vi "ChangeConfigGUI.vi"(4 "error in (no error)":errorcluster, 5 "Configuration Flags":T3, 6 "Configuration Read":T4 {"Select Mode:" items=["Custom", "Imaging", "300 All", "600 UV", "600 Blue", "600 Mid", "600 Red", "1200 m0", "1200 m1", "1200 m2", "1200 m3", "1200 m4", "1200 m5", "1200 m6", "1200 m7", "1200 RESOLVE", "400 m1", "400 m2", "930 m1", "930 m2", "930 m3", "930 m4", "930 m5", "930 m6", "400KL"]}, 7 "Alt Cam Focus":i32) -> (0 "error out":errorcluster, 1 "Script":T1[](array[typedef]), 2 "Targets":T2 {"Select Mode:" items=["Custom", "Imaging", "300 All", "600 UV", "600 Blue", "600 Mid", "600 Red", "1200 m0", "1200 m1", "1200 m2", "1200 m3", "1200 m4", "1200 m5", "1200 m6", "1200 m7", "1200 RESOLVE", "400 m1", "400 m2", "930 m1", "930 m2", "930 m3", "930 m4", "930 m5", "930 m6", "400KL"]})   [LabVIEW 2015]
doc: "This GUI interprets supplied configuration information and displays it to the user. It compares the target configuration to the machine state (what components are loaded) and checks for compatibility. If the user choses to start a move, an enumerated script is output that can be used to start a sequence of moves."
uses:
  GSP_ObsConfig.llb/configuration.ctl
  Script_actions.ctl
  Users/Stephen/Desktop/BETA_GSCS - Copy/Dialog/dialog_messages.ctl
  Users/Stephen/Desktop/BETA_GSCS - Copy/GUI/GSP_GUI_global.vi
panel:
  in  "Something not loaded?":bool
  out "Date":string
  out "User":string
  out "Name":string
  in  "Start Move":bool
  in  "Configuration":i32(listbox)
  # "Systems will finish any current scripts \nbefore beginning the configuration\nchange."
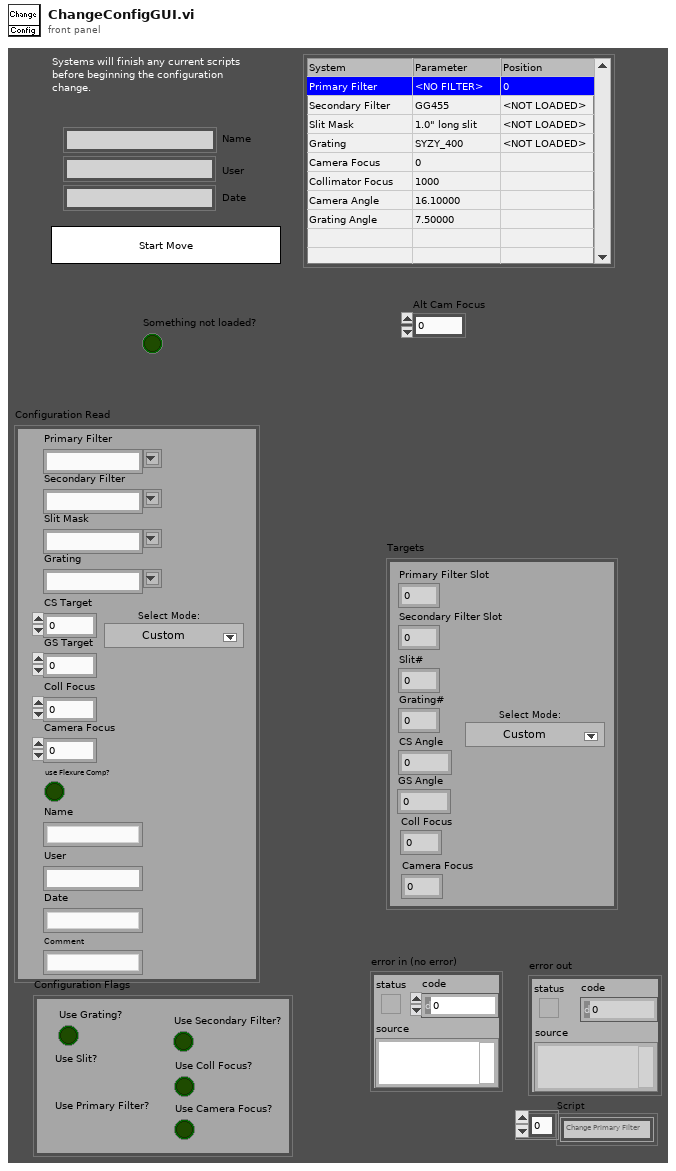
[diagram p1: front panel]
types:
  T1 = typedef "Script_actions.ctl" = enum16{"Change Primary Filter", "Change Secondary Filter", "Change Collimator Focus", "Change Camera Focus", "Change Grating", "Change Angles", "Change Slit Mask", "Toggle Slit", "Change WAVMODE", "Check All Systems", "Change Flexure"}
  T2 = cluster{"Primary Filter Slot":i32, "Secondary Filter Slot":i32, "Slit#":i32, "Grating#":i32, "CS Angle":dbl, "GS Angle":dbl, "Coll Focus":i32, "Camera Focus":i32, "Select Mode:":u16}
  T3 = cluster{"Use Grating?":bool, "Use Slit?":bool, "Use Primary Filter?":bool, "Use Secondary Filter?":bool, "Use Coll Focus?":bool, "Use Camera Focus?":bool}
  T4 = typedef "configuration.ctl" = cluster{"Primary Filter":string, "Secondary Filter":string, "Slit Mask":string, "Grating":string, "CS Target":dbl, "GS Target":dbl, "Coll Focus":i32, "Camera Focus":i32, "Name":string, "User":string, "Date":string, "Comment":string, "use Flexure Comp?":bool, "Select Mode:":u16}
  T5 = cluster{"Primary Filter Slot":i32, "Secondary Filter Slot":i32, "Slit#":i32, "Grating#":i32, "CS Angle":dbl, "GS Angle":dbl, "Coll Focus":i32, "Camera Focus":i32, "Select Mode":i32}
  T6 = typedef "dialog_messages.ctl" = enum16{"Custom", "Incompatible Config"}
  T7 = cluster{"Grating#":i32, "Slit#":i32, "Primary Filter#":i32, "Secondary Filter#":i32, "Coll Position":i32, "Camera Focus":i32, "Camera Angle":dbl, "Grating Angle":dbl, "Coll Temp":dbl, "CF Temp\n":dbl, "Camera Target":dbl, "Grating Target":dbl, "WAVMODE":string, "Slit Hidden??":bool}
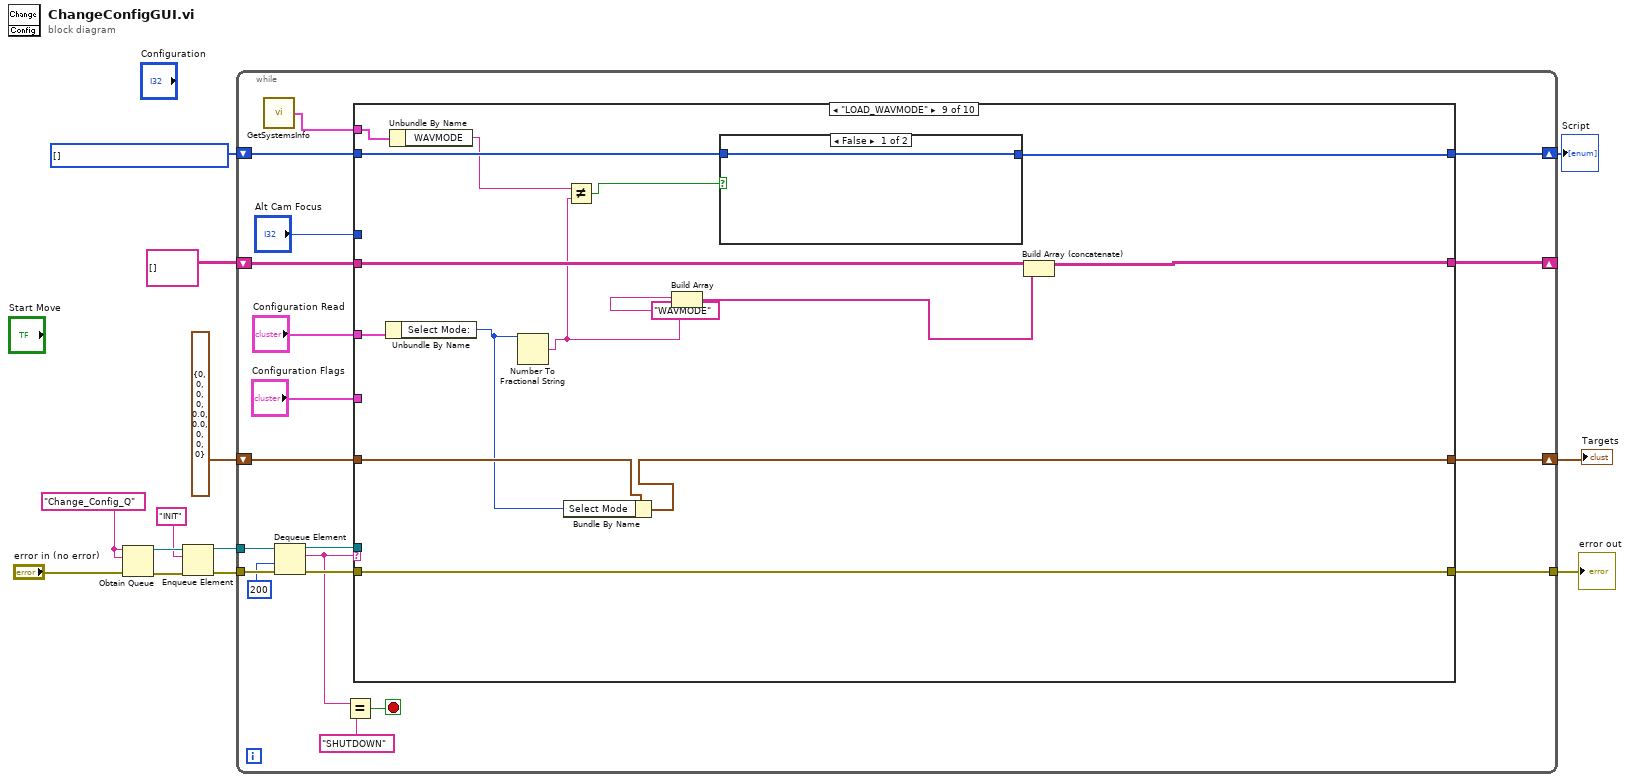
[diagram p0: block diagram]
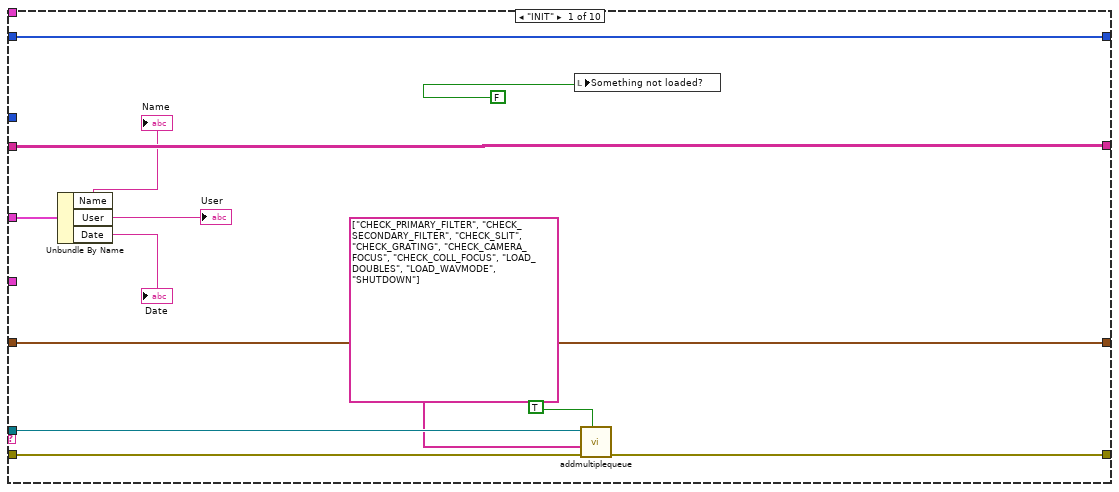
[diagram p2: hidden frame]
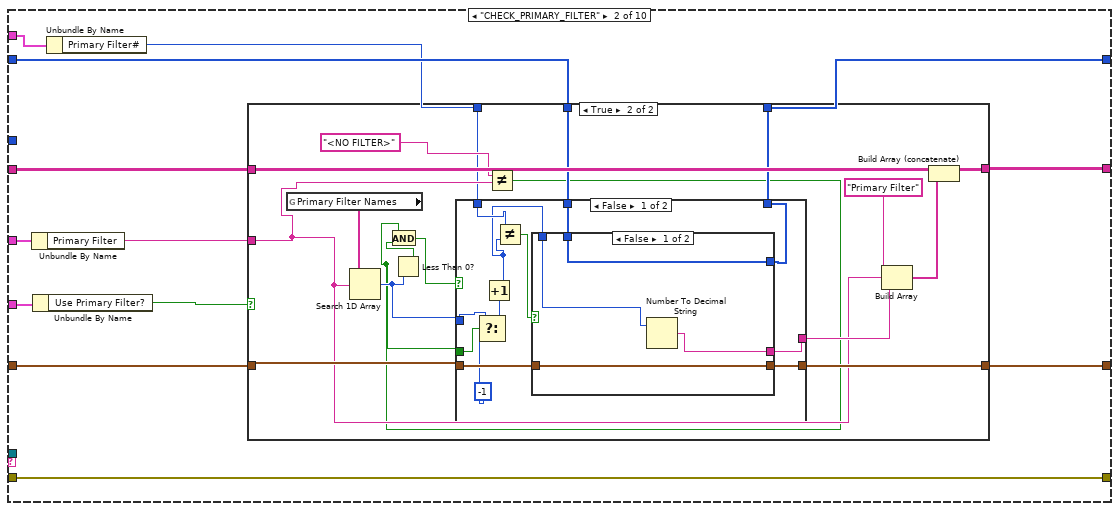
[diagram p3: hidden frame]
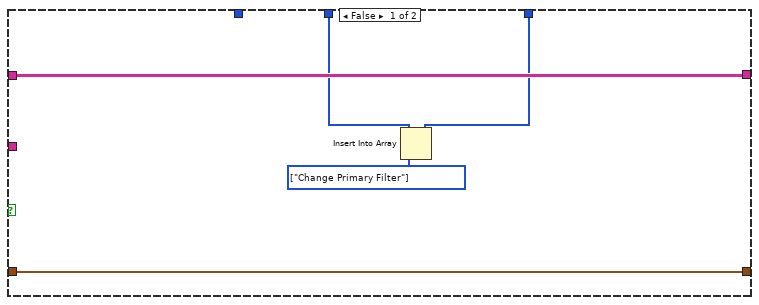
[diagram p4: hidden frame]
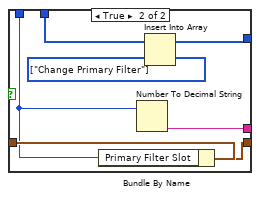
[diagram p5: hidden frame]
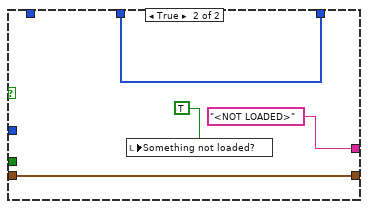
[diagram p6: hidden frame]
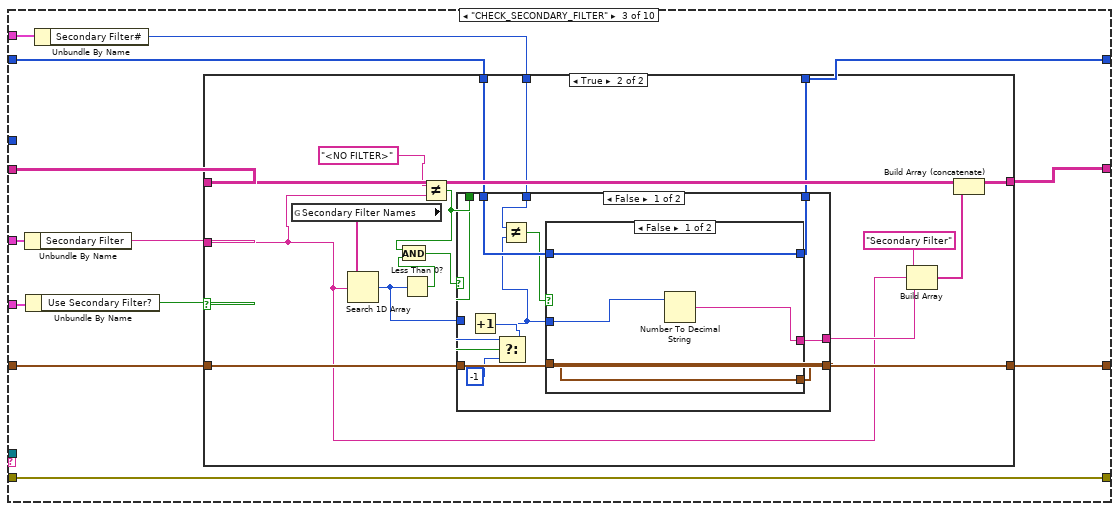
[diagram p7: hidden frame]
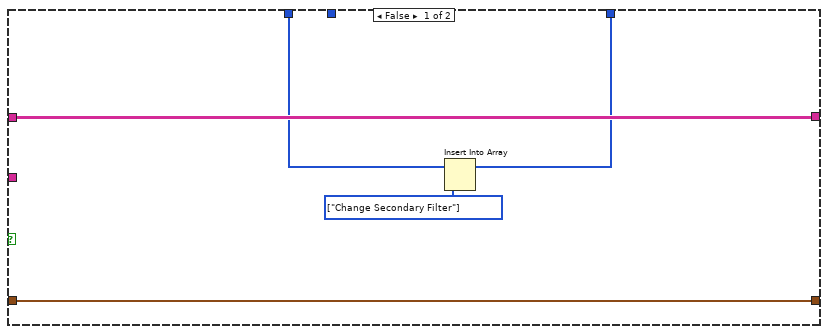
[diagram p8: hidden frame]
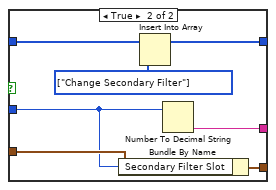
[diagram p9: hidden frame]
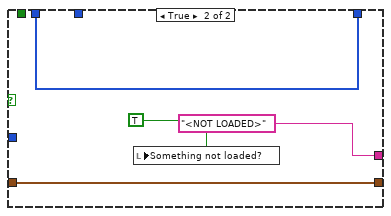
[diagram p10: hidden frame]
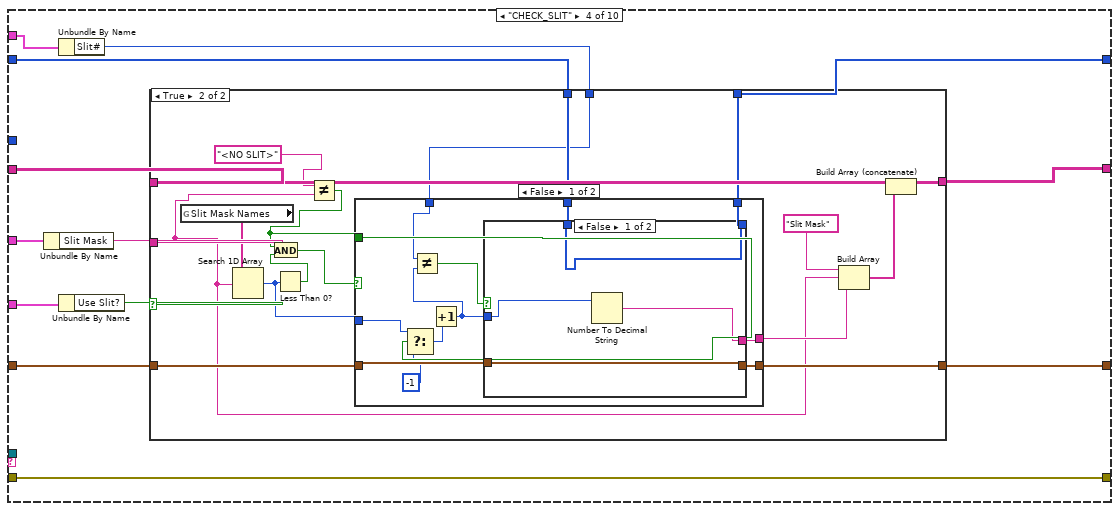
[diagram p11: hidden frame]
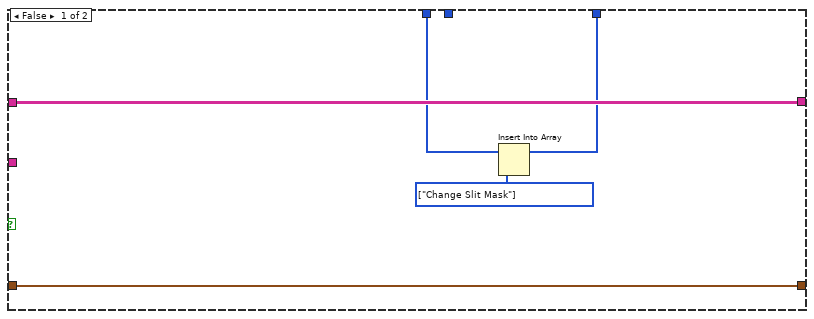
[diagram p12: hidden frame]
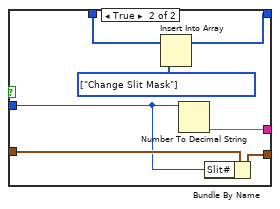
[diagram p13: hidden frame]
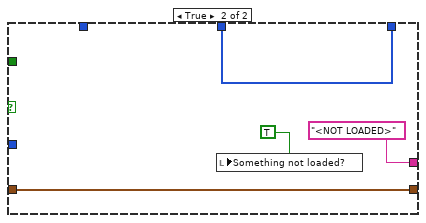
[diagram p14: hidden frame]
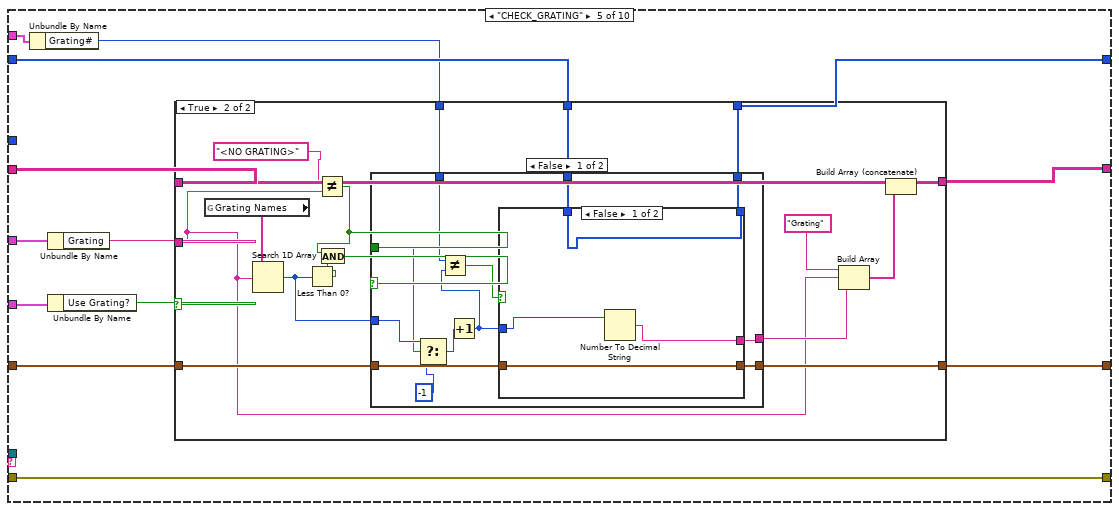
[diagram p15: hidden frame]
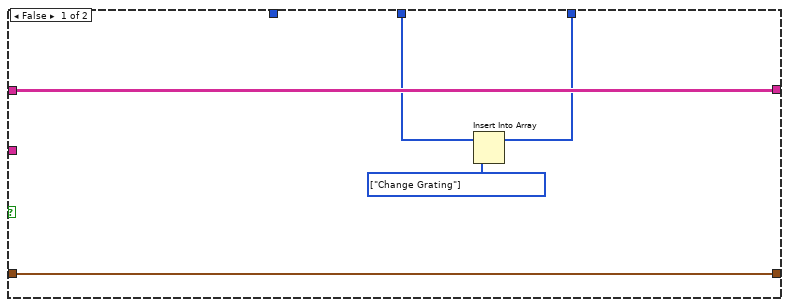
[diagram p16: hidden frame]
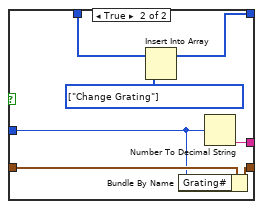
[diagram p17: hidden frame]
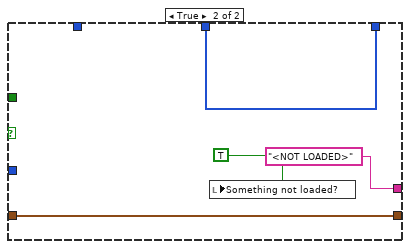
[diagram p18: hidden frame]
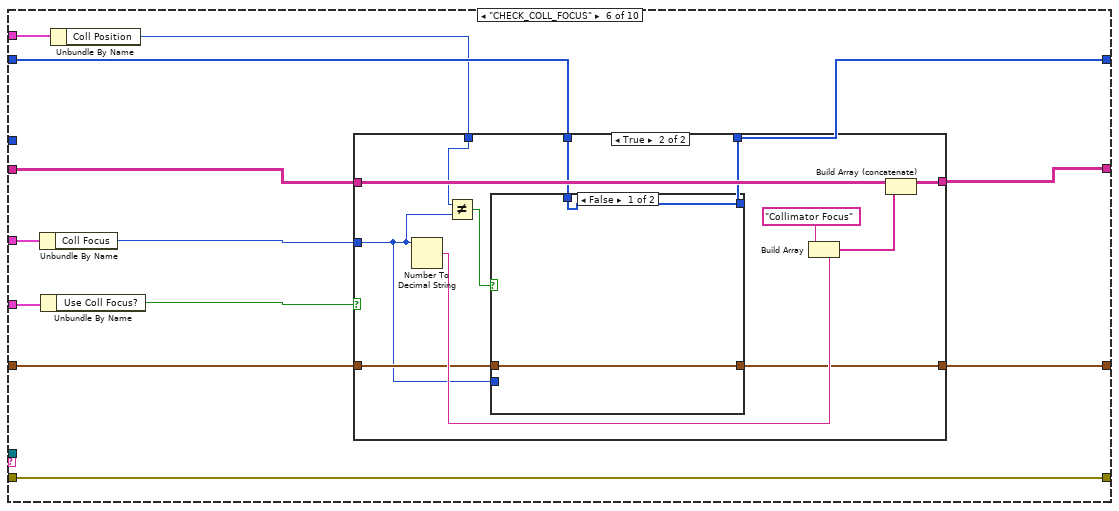
[diagram p19: hidden frame]
diagram:
  w4 = T1[] [] items=["Change Primary Filter", "Change Secondary Filter", "Change Collimator Focus", "Change Camera Focus", "Change Grating", "Change Angles", "Change Slit Mask", "Toggle Slit", "Change WAVMODE", "Check All Systems", "Change Flexure"]
  w11 = "Change_Config_Q" ("name (unnamed)")
  n1 = Obtain Queue(name (unnamed)=w11, element data type=w11, error in (no error)="error in (no error)") -> (queue out=w8:refnum<queue>, error out=w9:errorcluster)  [unwired: 2 in, 1 out]
  n2 = Enqueue Element(queue=w8, element="INIT", error in (no error)=w9) -> (queue out=w7:refnum<queue>, error out=w10:errorcluster)  [unwired: 1 in, 1 out]
  n3 = while {
    tunnel: w10 -> [w31]
    tunnel: [w32] -> w13
    tunnel: w7 -> [w29]
    shift-right: [w22] -> _
    shift-left: string[][] [] -> [w23]
    shift-right: [w18] -> w1
    shift-left: w4 -> [w19]
    shift-right: [w16] -> w2
    shift-left: T5 {"Primary Filter Slot"=0, "Secondary Filter Slot"=0, "Slit#"=0, "Grating#"=0, "CS Angle"=0.0, "GS Angle"=0.0, "Coll Focus"=0, "Camera Focus"=0, "Select Mode"=0} ("Targets") -> [w17]
    stop <- w25 stop-if-true
    n4 = call "GetSystemsInfo.vi"() -> ("Pos Info"=w14:T7)
    n5 = Dequeue Element(queue=w29, timeout in ms (-1)=200, error in (no error)=w31) -> (queue out=w28:refnum<queue>, element=w27:string, error out=w30:errorcluster)  [unwired: 1 out]
    n6 = Equal?(x=w27, y="SHUTDOWN") -> (x = y?=w25:bool)
    n7 = case shown="\"LOAD_WAVMODE\"" w27 {
      tunnel: w30 -> [w40 w52 w114 w176 w238 w300 w340 w383 w427 w440]
      tunnel: [w38 w52 w114 w176 w238 w300 w340 w377 w427 w440] -> w32
      tunnel: w28 -> [w39 _ _ _ _ _ _ _ _ _]
      tunnel: w23 -> [w45 w56 w118 w180 w242 w304 w343 w391 w432 w439]
      tunnel: [w45 w53 w115 w177 w239 w301 w341 w382 w430 w439] -> w22
      tunnel: "Configuration Read" -> [w44 w58 w120 w182 w244 w306 w345 w386 w425 _]
      tunnel: "Configuration Flags" -> [_ w57 w119 w181 w243 w305 w344 _ _ _]
      tunnel: w19 -> [w36 w51 w113 w175 w237 w299 w339 w381 w429 w437]
      tunnel: [w36 w50 w112 w174 w236 w298 w338 w380 w428 w437] -> w18
      tunnel: w17 -> [w35 w49 w111 w173 w235 w297 w337 w385 w424 w438]
      tunnel: [w35 w48 w110 w172 w234 w296 w336 w384 w423 w438] -> w16
      tunnel: "Alt Cam Focus" -> [_ _ _ _ _ _ w333 _ _ _]
      tunnel: w14 -> [_ w47 w109 w171 w233 w295 w331 w376 w421 _]
      frame "INIT" {
        n8 = Unbundle By Name(w44) -> ("Name"=→"Name":string, "User"=→"User":string, "Date"=→"Date":string)
        n9 = local write "Something not loaded?"(FALSE) -> ()
        n10 = call "addmultiplequeue.vi"("Add All (false)"=TRUE, "error in (no error)"=w40, "Strings to Add"=string[] ["CHECK_PRIMARY_FILTER", "CHECK_SECONDARY_FILTER", "CHECK_SLIT", "CHECK_GRATING", "CHECK_CAMERA_FOCUS", "CHECK_COLL_FOCUS", "LOAD_DOUBLES", "LOAD_WAVMODE", "SHUTDOWN"], "queue"=w39) -> ("error out"=w38:errorcluster)  [unwired: 3 in, 1 out]
      }
      frame "CHECK_PRIMARY_FILTER" {
        n11 = Unbundle By Name(w58) -> ("Primary Filter"=w54:string)
        n12 = Unbundle By Name(w57) -> ("Use Primary Filter?"=w55:bool)
        n13 = Unbundle By Name(w47) -> ("Primary Filter#"=w46:i32)
        n14 = case shown="True" w55 {
          tunnel: w56 -> [w63 w77]
          tunnel: w54 -> [_ w68]
          tunnel: [w63 w78] -> w53
          tunnel: w51 -> [w62 w73]
          tunnel: [w61 w72] -> w50
          tunnel: w49 -> [w60 w71]
          tunnel: [w60 w70] -> w48
          tunnel: w46 -> [_ w64]
          frame False {
            w59 = T1[] [enum."Change Primary Filter"] items=["Change Primary Filter", "Change Secondary Filter", "Change Collimator Focus", "Change Camera Focus", "Change Grating", "Change Angles", "Change Slit Mask", "Toggle Slit", "Change WAVMODE", "Check All Systems", "Change Flexure"]
            n15 = Insert Into Array(array=w62, new element=w59) -> (w61:T1[])  [unwired: 1 in]
          }
          frame True {
            n16 = global read "GSP_GUI_global.vi" "Primary Filter Names"() -> (w80:string[])
            n17 = Search 1D Array(1D array=w80, element=w68) -> (index of element=w79:i32)  [unwired: 1 in]
            n18 = Less Than 0?(x=w79) -> (x < 0?=w67:bool)
            n19 = Not Equal?(x="<NO FILTER>", y=w68) -> (x != y?=w65:bool)
            n20 = And(x=w65, y=w67) -> (x .and. y?=w66:bool)
            n21 = case shown="False" w66 {
              tunnel: w79 -> [w86 _]
              tunnel: [w92 "<NOT LOADED>"] -> w75
              tunnel: w73 -> [w91 w106]
              tunnel: [w90 w106] -> w72
              tunnel: w71 -> [w89 w105]
              tunnel: [w88 w105] -> w70
              tunnel: w65 -> [w84 _]
              tunnel: w64 -> [w83 _]
              frame False {
                n22 = Select(t=w86, s=w84, f=-1) -> (s? t:f=w85:i32)
                n23 = Increment(x=w85) -> (x+1=w81:i32)
                n24 = Not Equal?(x=w83, y=w81) -> (x != y?=w82:bool)
                n25 = case shown="False" w82 {
                  tunnel: [w93 w103] -> w92
                  tunnel: w91 -> [w96 w102]
                  tunnel: [w96 w101] -> w90
                  tunnel: w89 -> [w95 w100]
                  tunnel: [w95 w99] -> w88
                  tunnel: w81 -> [w94 w98]
                  frame False {
                    n26 = Number To Decimal String(number=w94) -> (decimal integer string=w93:string)  [unwired: 1 in]
                  }
                  frame True {
                    w97 = T1[] [enum."Change Primary Filter"] items=["Change Primary Filter", "Change Secondary Filter", "Change Collimator Focus", "Change Camera Focus", "Change Grating", "Change Angles", "Change Slit Mask", "Toggle Slit", "Change WAVMODE", "Check All Systems", "Change Flexure"]
                    n27 = Bundle By Name(cluster=w100, "Primary Filter Slot"=w98) -> (w99:T5)
                    n28 = Number To Decimal String(number=w98) -> (decimal integer string=w103:string)  [unwired: 1 in]
                    n29 = Insert Into Array(array=w102, new element=w97) -> (w101:T1[])  [unwired: 1 in]
                  }
                }
              }
              frame True {
                n30 = local write "Something not loaded?"(TRUE) -> ()
              }
            }
            n31 = Build Array("Primary Filter", w68, w75) -> (w74:string[])
            n32 = Build Array (concatenate)(w77, w74) -> (w78:string[][])
          }
        }
      }
      frame "CHECK_SECONDARY_FILTER" {
        n33 = Unbundle By Name(w120) -> ("Secondary Filter"=w116:string)
        n34 = Unbundle By Name(w119) -> ("Use Secondary Filter?"=w117:bool)
        n35 = Unbundle By Name(w109) -> ("Secondary Filter#"=w108:i32)
        n36 = case shown="True" w117 {
          tunnel: w118 -> [w125 w139]
          tunnel: w116 -> [_ w130]
          tunnel: [w125 w140] -> w115
          tunnel: w113 -> [w124 w135]
          tunnel: [w123 w134] -> w112
          tunnel: w111 -> [w122 w133]
          tunnel: [w122 w132] -> w110
          tunnel: w108 -> [_ w126]
          frame False {
            w121 = T1[] [enum."Change Secondary Filter"] items=["Change Primary Filter", "Change Secondary Filter", "Change Collimator Focus", "Change Camera Focus", "Change Grating", "Change Angles", "Change Slit Mask", "Toggle Slit", "Change WAVMODE", "Check All Systems", "Change Flexure"]
            n37 = Insert Into Array(array=w124, new element=w121) -> (w123:T1[])  [unwired: 1 in]
          }
          frame True {
            n38 = global read "GSP_GUI_global.vi" "Secondary Filter Names"() -> (w142:string[])
            n39 = Search 1D Array(1D array=w142, element=w130) -> (index of element=w141:i32)  [unwired: 1 in]
            n40 = Less Than 0?(x=w141) -> (x < 0?=w129:bool)
            n41 = Not Equal?(x="<NO FILTER>", y=w130) -> (x != y?=w127:bool)
            n42 = And(x=w127, y=w129) -> (x .and. y?=w128:bool)
            n43 = case shown="False" w128 {
              tunnel: w141 -> [w148 _]
              tunnel: [w154 "<NOT LOADED>"] -> w137
              tunnel: w135 -> [w153 w168]
              tunnel: [w152 w168] -> w134
              tunnel: w133 -> [w151 w167]
              tunnel: [w150 w167] -> w132
              tunnel: w127 -> [w146 _]
              tunnel: w126 -> [w145 _]
              frame False {
                n44 = Select(t=w148, s=w146, f=-1) -> (s? t:f=w147:i32)
                n45 = Increment(x=w147) -> (x+1=w144:i32)
                n46 = Not Equal?(x=w145, y=w144) -> (x != y?=w143:bool)
                n47 = case shown="False" w143 {
                  tunnel: [w157 w165] -> w154
                  tunnel: w153 -> [w155 w164]
                  tunnel: [w155 w163] -> w152
                  tunnel: w151 -> [w156 w162]
                  tunnel: [w156 w161] -> w150
                  tunnel: w144 -> [w158 w160]
                  frame False {
                    n48 = Number To Decimal String(number=w158) -> (decimal integer string=w157:string)  [unwired: 1 in]
                  }
                  frame True {
                    w159 = T1[] [enum."Change Secondary Filter"] items=["Change Primary Filter", "Change Secondary Filter", "Change Collimator Focus", "Change Camera Focus", "Change Grating", "Change Angles", "Change Slit Mask", "Toggle Slit", "Change WAVMODE", "Check All Systems", "Change Flexure"]
                    n49 = Bundle By Name(cluster=w162, "Secondary Filter Slot"=w160) -> (w161:T5)
                    n50 = Insert Into Array(array=w164, new element=w159) -> (w163:T1[])  [unwired: 1 in]
                    n51 = Number To Decimal String(number=w160) -> (decimal integer string=w165:string)  [unwired: 1 in]
                  }
                }
              }
              frame True {
                n52 = local write "Something not loaded?"(TRUE) -> ()
              }
            }
            n53 = Build Array("Secondary Filter", w130, w137) -> (w136:string[])
            n54 = Build Array (concatenate)(w139, w136) -> (w140:string[][])
          }
        }
      }
      frame "CHECK_SLIT" {
        n55 = Unbundle By Name(w182) -> ("Slit Mask"=w178:string)
        n56 = Unbundle By Name(w171) -> ("Slit#"=w170:i32)
        n57 = Unbundle By Name(w181) -> ("Use Slit?"=w179:bool)
        n58 = case shown="True" w179 {
          tunnel: w180 -> [w187 w201]
          tunnel: w178 -> [_ w192]
          tunnel: [w187 w202] -> w177
          tunnel: w175 -> [w186 w197]
          tunnel: [w185 w196] -> w174
          tunnel: w173 -> [w184 w195]
          tunnel: [w184 w194] -> w172
          tunnel: w170 -> [_ w188]
          frame False {
            w183 = T1[] [enum."Change Slit Mask"] items=["Change Primary Filter", "Change Secondary Filter", "Change Collimator Focus", "Change Camera Focus", "Change Grating", "Change Angles", "Change Slit Mask", "Toggle Slit", "Change WAVMODE", "Check All Systems", "Change Flexure"]
            n59 = Insert Into Array(array=w186, new element=w183) -> (w185:T1[])  [unwired: 1 in]
          }
          frame True {
            n60 = global read "GSP_GUI_global.vi" "Slit Mask Names"() -> (w204:string[])
            n61 = Search 1D Array(1D array=w204, element=w192) -> (index of element=w203:i32)  [unwired: 1 in]
            n62 = Less Than 0?(x=w203) -> (x < 0?=w191:bool)
            n63 = Not Equal?(x="<NO SLIT>", y=w192) -> (x != y?=w189:bool)
            n64 = And(x=w189, y=w191) -> (x .and. y?=w190:bool)
            n65 = case shown="False" w190 {
              tunnel: w203 -> [w211 _]
              tunnel: [w216 "<NOT LOADED>"] -> w199
              tunnel: w197 -> [w215 w230]
              tunnel: [w214 w230] -> w196
              tunnel: w195 -> [w213 w229]
              tunnel: [w212 w229] -> w194
              tunnel: w189 -> [w210 _]
              tunnel: w188 -> [w206 _]
              frame False {
                n66 = Select(t=w211, s=w210, f=-1) -> (s? t:f=w208:i32)
                n67 = Increment(x=w208) -> (x+1=w207:i32)
                n68 = Not Equal?(x=w206, y=w207) -> (x != y?=w205:bool)
                n69 = case shown="False" w205 {
                  tunnel: [w219 w227] -> w216
                  tunnel: w215 -> [w217 w226]
                  tunnel: [w217 w225] -> w214
                  tunnel: w213 -> [w218 w224]
                  tunnel: [w218 w223] -> w212
                  tunnel: w207 -> [w220 w222]
                  frame False {
                    n70 = Number To Decimal String(number=w220) -> (decimal integer string=w219:string)  [unwired: 1 in]
                  }
                  frame True {
                    w221 = T1[] [enum."Change Slit Mask"] items=["Change Primary Filter", "Change Secondary Filter", "Change Collimator Focus", "Change Camera Focus", "Change Grating", "Change Angles", "Change Slit Mask", "Toggle Slit", "Change WAVMODE", "Check All Systems", "Change Flexure"]
                    n71 = Insert Into Array(array=w226, new element=w221) -> (w225:T1[])  [unwired: 1 in]
                    n72 = Number To Decimal String(number=w222) -> (decimal integer string=w227:string)  [unwired: 1 in]
                    n73 = Bundle By Name(cluster=w224, "Slit#"=w222) -> (w223:T5)
                  }
                }
              }
              frame True {
                n74 = local write "Something not loaded?"(TRUE) -> ()
              }
            }
            n75 = Build Array("Slit Mask", w192, w199) -> (w198:string[])
            n76 = Build Array (concatenate)(w201, w198) -> (w202:string[][])
          }
        }
      }
      frame "CHECK_GRATING" {
        n77 = Unbundle By Name(w233) -> ("Grating#"=w232:i32)
        n78 = Unbundle By Name(w244) -> ("Grating"=w240:string)
        n79 = Unbundle By Name(w243) -> ("Use Grating?"=w241:bool)
        n80 = case shown="True" w241 {
          tunnel: w242 -> [w249 w263]
          tunnel: w240 -> [_ w253]
          tunnel: [w249 w264] -> w239
          tunnel: w237 -> [w248 w259]
          tunnel: [w247 w258] -> w236
          tunnel: w235 -> [w246 w257]
          tunnel: [w246 w256] -> w234
          tunnel: w232 -> [_ w250]
          frame False {
            w245 = T1[] [enum."Change Grating"] items=["Change Primary Filter", "Change Secondary Filter", "Change Collimator Focus", "Change Camera Focus", "Change Grating", "Change Angles", "Change Slit Mask", "Toggle Slit", "Change WAVMODE", "Check All Systems", "Change Flexure"]
            n81 = Insert Into Array(array=w248, new element=w245) -> (w247:T1[])  [unwired: 1 in]
          }
          frame True {
            n82 = global read "GSP_GUI_global.vi" "Grating Names"() -> (w266:string[])
            n83 = Search 1D Array(1D array=w266, element=w253) -> (index of element=w265:i32)  [unwired: 1 in]
            n84 = Less Than 0?(x=w265) -> (x < 0?=w255:bool)
            n85 = Not Equal?(x="<NO GRATING>", y=w253) -> (x != y?=w251:bool)
            n86 = And(x=w251, y=w255) -> (x .and. y?=w254:bool)
            n87 = case shown="False" w254 {
              tunnel: w265 -> [w272 _]
              tunnel: [w278 "<NOT LOADED>"] -> w261
              tunnel: w259 -> [w277 w292]
              tunnel: [w276 w292] -> w258
              tunnel: w257 -> [w275 w291]
              tunnel: [w274 w291] -> w256
              tunnel: w251 -> [w270 _]
              tunnel: w250 -> [w267 _]
              frame False {
                n88 = Select(t=w272, s=w270, f=-1) -> (s? t:f=w271:i32)
                n89 = Increment(x=w271) -> (x+1=w268:i32)
                n90 = Not Equal?(x=w267, y=w268) -> (x != y?=w269:bool)
                n91 = case shown="False" w269 {
                  tunnel: [w279 w289] -> w278
                  tunnel: w277 -> [w282 w288]
                  tunnel: [w282 w287] -> w276
                  tunnel: w275 -> [w281 w286]
                  tunnel: [w281 w285] -> w274
                  tunnel: w268 -> [w280 w284]
                  frame False {
                    n92 = Number To Decimal String(number=w280) -> (decimal integer string=w279:string)  [unwired: 1 in]
                  }
                  frame True {
                    w283 = T1[] [enum."Change Grating"] items=["Change Primary Filter", "Change Secondary Filter", "Change Collimator Focus", "Change Camera Focus", "Change Grating", "Change Angles", "Change Slit Mask", "Toggle Slit", "Change WAVMODE", "Check All Systems", "Change Flexure"]
                    n93 = Insert Into Array(array=w288, new element=w283) -> (w287:T1[])  [unwired: 1 in]
                    n94 = Bundle By Name(cluster=w286, "Grating#"=w284) -> (w285:T5)
                    n95 = Number To Decimal String(number=w284) -> (decimal integer string=w289:string)  [unwired: 1 in]
                  }
                }
              }
              frame True {
                n96 = local write "Something not loaded?"(TRUE) -> ()
              }
            }
            n97 = Build Array("Grating", w253, w261) -> (w260:string[])
            n98 = Build Array (concatenate)(w263, w260) -> (w264:string[][])
          }
        }
      }
      frame "CHECK_COLL_FOCUS" {
        n99 = Unbundle By Name(w306) -> ("Coll Focus"=w302:i32)
        n100 = Unbundle By Name(w305) -> ("Use Coll Focus?"=w303:bool)
        n101 = Unbundle By Name(w295) -> ("Coll Position"=w294:i32)
        n102 = case shown="True" w303 {
          tunnel: w304 -> [w309 w320]
          tunnel: w302 -> [_ w311]
          tunnel: [w309 w321] -> w301
          tunnel: w299 -> [w307 w317]
          tunnel: [w307 w316] -> w298
          tunnel: w297 -> [w308 w314]
          tunnel: [w308 w313] -> w296
          tunnel: w294 -> [_ w312]
          frame False {
          }
          frame True {
            n103 = Number To Decimal String(number=w311) -> (decimal integer string=w315:string)  [unwired: 1 in]
            n104 = Not Equal?(x=w312, y=w311) -> (x != y?=w310:bool)
            n105 = case shown="False" w310 {
              tunnel: w317 -> [w323 w329]
              tunnel: [w323 w328] -> w316
              tunnel: w314 -> [w322 w327]
              tunnel: w311 -> [_ w326]
              tunnel: [w322 w325] -> w313
              frame False {
              }
              frame True {
                w324 = T1[] [enum."Change Collimator Focus"] items=["Change Primary Filter", "Change Secondary Filter", "Change Collimator Focus", "Change Camera Focus", "Change Grating", "Change Angles", "Change Slit Mask", "Toggle Slit", "Change WAVMODE", "Check All Systems", "Change Flexure"]
                n106 = Bundle By Name(cluster=w327, "Coll Focus"=w326) -> (w325:T5)
                n107 = Insert Into Array(array=w329, new element=w324) -> (w328:T1[])  [unwired: 1 in]
              }
            }
            n108 = Build Array("Collimator Focus", w315) -> (w318:string[])
            n109 = Build Array (concatenate)(w320, w318) -> (w321:string[][])
          }
        }
      }
      frame "CHECK_CAMERA_FOCUS" {
        n110 = Not Equal To 0?(x=w333) -> (x != 0?=w334:bool)
        n111 = Unbundle By Name(w345) -> ("Camera Focus"=w335:i32)
        n112 = Unbundle By Name(w344) -> ("Use Camera Focus?"=w342:bool)
        n113 = Unbundle By Name(w331) -> ("Camera Focus"=w330:i32)
        n114 = Select(t=w333, s=w334, f=w335) -> (s? t:f=w332:i32)
        n115 = case shown="True" w342 {
          tunnel: w343 -> [w348 w359]
          tunnel: w332 -> [_ w351]
          tunnel: [w348 w360] -> w341
          tunnel: w339 -> [w346 w356]
          tunnel: [w346 w355] -> w338
          tunnel: w337 -> [w347 w353]
          tunnel: [w347 w352] -> w336
          tunnel: w330 -> [_ w349]
          frame False {
          }
          frame True {
            n116 = Not Equal?(x=w349, y=w351) -> (x != y?=w350:bool)
            n117 = Number To Decimal String(number=w351) -> (decimal integer string=w354:string)  [unwired: 1 in]
            n118 = case shown="False" w350 {
              tunnel: w356 -> [w361 w368]
              tunnel: [w361 w367] -> w355
              tunnel: w353 -> [w362 w366]
              tunnel: w351 -> [_ w365]
              tunnel: [w362 w364] -> w352
              frame False {
              }
              frame True {
                w363 = T1[] [enum."Change Camera Focus"] items=["Change Primary Filter", "Change Secondary Filter", "Change Collimator Focus", "Change Camera Focus", "Change Grating", "Change Angles", "Change Slit Mask", "Toggle Slit", "Change WAVMODE", "Check All Systems", "Change Flexure"]
                n119 = Bundle By Name(cluster=w366, "Camera Focus"=w365) -> (w364:T5)
                n120 = Insert Into Array(array=w368, new element=w363) -> (w367:T1[])  [unwired: 1 in]
              }
            }
            n121 = Build Array("Camera Focus", w354) -> (w357:string[])
            n122 = Build Array (concatenate)(w359, w357) -> (w360:string[][])
          }
        }
      }
      frame "LOAD_DOUBLES" {
        n123 = Unbundle By Name(w376) -> ("Camera Angle"=w373:dbl, "Grating Angle"=w371:dbl)
        n124 = Unbundle By Name(w386) -> ("CS Target"=w372:dbl, "GS Target"=w370:dbl)
        n125 = Not Equal?(x=w373, y=w372) -> (x != y?=w374:bool)
        n126 = Not Equal?(x=w371, y=w370) -> (x != y?=w375:bool)
        n127 = Number To Fractional String(number=w372, precision (6)=i16 5) -> (F-format string=w388:string)  [unwired: 2 in]
        n128 = Number To Fractional String(number=w370, precision (6)=i16 5) -> (F-format string=w387:string)  [unwired: 2 in]
        n129 = Bundle By Name(cluster=w385, "CS Angle"=w372, "GS Angle"=w370) -> (w384:T5)
        n130 = Or(x=w374, y=w375) -> (x .or. y?=w369:bool)
        n131 = case shown="False" w369 {
          tunnel: w391 -> [w394 w413]
          tunnel: w388 -> [w393 w411]
          tunnel: w387 -> [w396 w409]
          tunnel: [w395 w405] -> w382
          tunnel: w381 -> [w401 w404]
          tunnel: [w401 w403] -> w380
          frame False {
            n132 = Build Array("Camera Angle", w393) -> (w399:string[])
            n133 = Build Array("Grating Angle", w396) -> (w398:string[])
            n134 = Build Array(w399, w398) -> (w397:string[][])
            n135 = Build Array (concatenate)(w394, w397) -> (w395:string[][])
          }
          frame True {
            w402 = T1[] [enum."Change Angles"] items=["Change Primary Filter", "Change Secondary Filter", "Change Collimator Focus", "Change Camera Focus", "Change Grating", "Change Angles", "Change Slit Mask", "Toggle Slit", "Change WAVMODE", "Check All Systems", "Change Flexure"]
            n136 = Build Array("Camera Angle", w411) -> (w408:string[])
            n137 = Build Array("Grating Angle", w409) -> (w407:string[])
            n138 = Build Array(w408, w407) -> (w406:string[][])
            n139 = Insert Into Array(array=w404, new element=w402) -> (w403:T1[])  [unwired: 1 in]
            n140 = Build Array (concatenate)(w413, w406) -> (w405:string[][])
          }
        }
        n141 = property on="Configuration" class="MCListbox (strict)"(error in=w383, "Item Names"=w382) -> (error out=w378:errorcluster)  [unwired: 1 in, 1 out]
        n142 = case shown="True" "Something not loaded?" {
          tunnel: w378 -> [w414 w417]
          tunnel: [w414 w415] -> w377
          frame False {
          }
          frame True {
            n143 = call "GSP_Dialog.vi"("error in (no error)"=w417, "Messages"=dialog_messages."Incompatible Config") -> ("error out"=w415:errorcluster)  [unwired: 5 in]
          }
        }
      }
      frame "LOAD_WAVMODE" {
        n144 = Unbundle By Name(w425) -> ("Select Mode:"=w422:u16)
        n145 = Unbundle By Name(w421) -> ("WAVMODE"=w420:string)
        n146 = Number To Fractional String(number=w422) -> (F-format string=w419:string)  [unwired: 3 in]
        n147 = Bundle By Name(cluster=w424, "Select Mode"=w422) -> (w423:T5)
        n148 = Not Equal?(x=w420, y=w419) -> (x != y?=w418:bool)
        n149 = Build Array("WAVMODE", w419) -> (w426:string[])
        n150 = case shown="False" w418 {
          tunnel: w429 -> [w433 w436]
          tunnel: [w433 w435] -> w428
          frame False {
          }
          frame True {
            w434 = T1[] [enum."Change WAVMODE"] items=["Change Primary Filter", "Change Secondary Filter", "Change Collimator Focus", "Change Camera Focus", "Change Grating", "Change Angles", "Change Slit Mask", "Toggle Slit", "Change WAVMODE", "Check All Systems", "Change Flexure"]
            n151 = Insert Into Array(array=w436, new element=w434) -> (w435:T1[])  [unwired: 1 in]
          }
        }
        n152 = Build Array (concatenate)(w432, w426) -> (w430:string[][])
      }
      frame "SHUTDOWN", Default {
      }
    }
  }
  "error out" <- w13
  "Targets" <- w2
  "Script" <- w1
